vi "ftt array.vi"(5 "Display":T1) -> (2 "appended array":string[](array[string]))   [LabVIEW 2014]
uses:
  Type'def/FTT Display Type.ctl
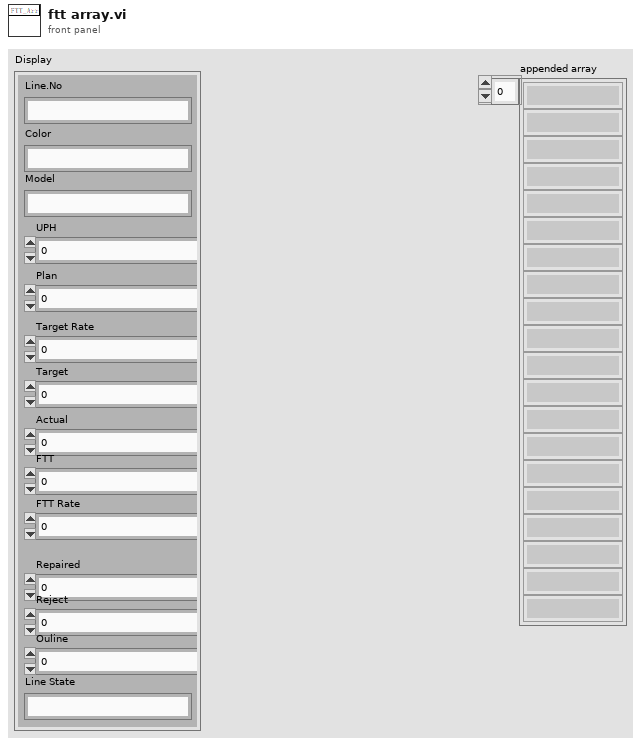
[diagram p1: front panel]
types:
  T1 = typedef "FTT Display Type.ctl" = cluster{"Line.No":string, "Model":string, "Color":string, "UPH":dbl, "Plan":dbl, "Target Rate":dbl, "Target ":dbl, "Actual":dbl, "FTT":dbl, "FTT Rate":dbl, "Repaired":dbl, "Reject":dbl, "Ouline":dbl, "Line State":string}
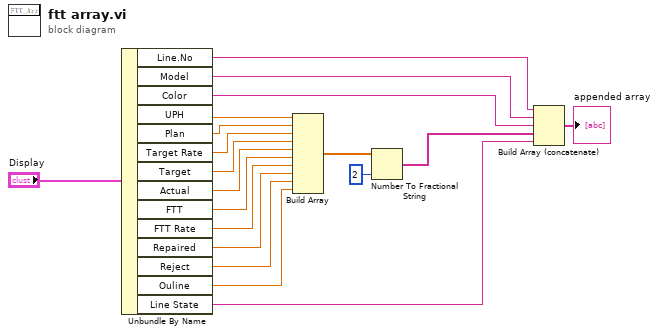
[diagram p0: block diagram]
diagram:
  n1 = Unbundle By Name("Display") -> ("Line.No"=w7:string, "Model"=w1:string, "Color"=w6:string, "UPH"=w18:dbl, "Plan"=w17:dbl, "Target Rate"=w16:dbl, "Target"=w15:dbl, "Actual"=w14:dbl, "FTT"=w13:dbl, "FTT Rate"=w12:dbl, "Repaired"=w11:dbl, "Reject"=w10:dbl, "Ouline"=w9:dbl, "Line State"=w4:string)
  n2 = Build Array(w18, w17, w16, w15, w14, w13, w12, w11, w10, w9) -> (w8:dbl[])
  n3 = Number To Fractional String(number=w8, precision (6)=i16 2) -> (F-format string=w5:string[])  [unwired: 2 in]
  n4 = Build Array (concatenate)(w7, w1, w6, w5, w4) -> (→"appended array":string[])
